vi "USS9804_InitAD.vi"(8 "Error In":errorcluster, 10 "para_init":T1, 11 "Handle":u64) -> (0 "Error Out":errorcluster, 3 "Handle 2":u64)   [LabVIEW 2015]
uses:
  para_init.ctl
  USS9804.DLL
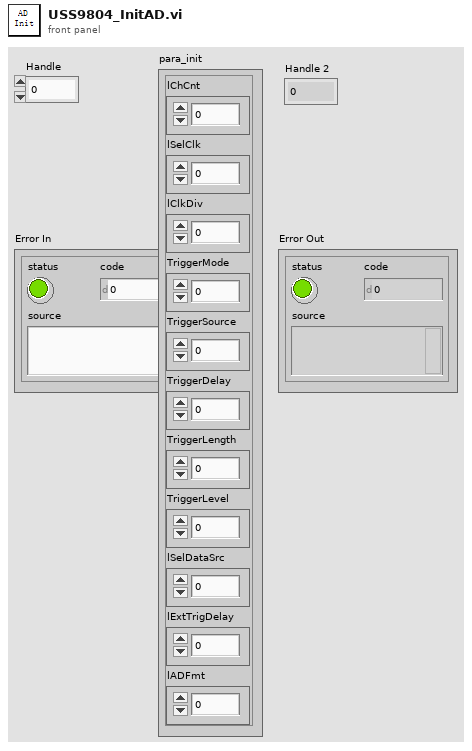
[diagram p1: front panel]
types:
  T1 = typedef "para_init.ctl" = cluster{"lChCnt":i32, "lSelClk":i32, "lClkDiv":i32, "TriggerMode":i32, "TriggerSource":i32, "TriggerDelay":i32, "TriggerLength":i32, "TriggerLevel":i32, "lSelDataSrc":i32, "lExtTrigDelay":i32, "lADFmt":i32}
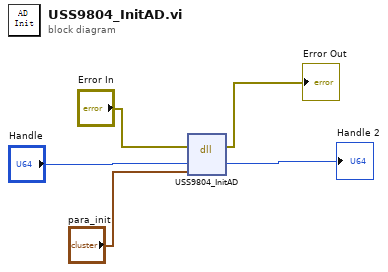
[diagram p0: block diagram]
diagram:
  n1 = dll-call lib="PTH2Sabs CYexinrongWorkplace\t普密斯Thickness-measurementLabVIEWUSS9804.DLL" fn="USS9804_InitAD"(error in="Error In", "Handle"="Handle", "para_init"="para_init") -> (error out=→"Error Out":errorcluster, "Handle"=→"Handle 2":u64)  [unwired: 4 in, 1 out]
